vi "Write Write Wvfms.vi"(8 "error in (no error)":errorcluster, 10 "Write Wvfms":bool, 11 "nPAS in":refnum<class "nPAS.lvclass">) -> (0 "error out":errorcluster, 3 "nPAS out":refnum<class "nPAS.lvclass">)   [LabVIEW 2018, in "gPAS Library.lvlib" / "nPAS.lvclass"]
uses:
  nPAS.lvclass
  nPAS.lvclass/nPAS.ctl
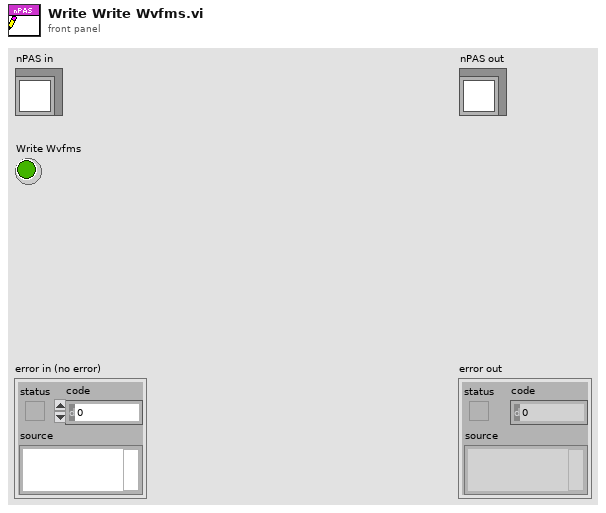
[diagram p1: front panel]
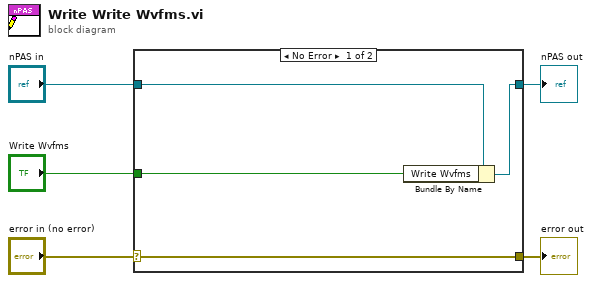
[diagram p0: block diagram]
diagram:
  n1 = case shown="No Error" "error in (no error)" {
    selector: "error in (no error)" -> [w9 w10]
    tunnel: [w9 w10] -> w4
    tunnel: [w7 w11] -> w2
    tunnel: "nPAS in" -> [w8 w11]
    tunnel: "Write Wvfms" -> [w6 _]
    frame No Error {
      n2 = Bundle By Name(cluster=w8, "Write Wvfms"=w6) -> (w7:refnum<class "nPAS.lvclass">)
    }
    frame Error {
    }
  }
  "error out" <- w4
  "nPAS out" <- w2
